vi "Ramp to Zero.vi"(8 "error in (no error)":errorcluster, 11 "Instrument.1820 in":refnum<class "Instrument.Oxford1820.lvclass">) -> (0 "error out":errorcluster, 2 "Response":string, 3 "Instrument.1820 in":refnum<class "Instrument.Oxford1820.lvclass">)   [LabVIEW 2016, in "Instrument.Oxford1820.lvclass"]
uses:
  Instrument.Oxford1820.lvclass
  <instrlib>/Mercury iXX/Public/Libraries/Magnet/Controls/PSU Actions.ctl
  Typedefs/Instrument.Oxford1820.Commands-enum.ctl
  <instrlib>/Mercury iXX/Public/Libraries/Magnet.lvlib
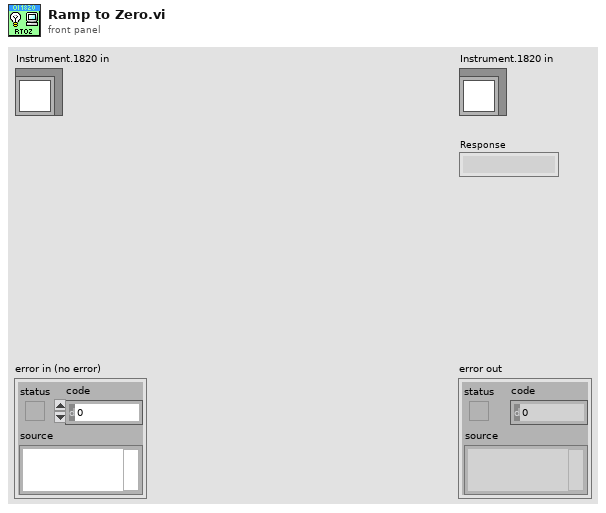
[diagram p1: front panel]
types:
  T1 = typedef "Instrument.Oxford1820.lvclass/Instrument.Oxford1820.Commands-enum.ctl" = enum16{"setAction", "setTarget", "setSwitchHeat", "setLambda", "setFillMode", "setNeedleValve", "setMagnetField", "getStatus", "getTarget", "getSwitchHeat", "getPSUField", "newcommand", "getMagnetField"}
  T2 = typedef "Mercury iXX.lvlib/Magnet.lvlib/PSU Actions.ctl" = string
  T3 = cluster{"Holding":bool, "Ramp to Setpoint":bool, "Ramp to Zero":bool, "Clamp":bool}
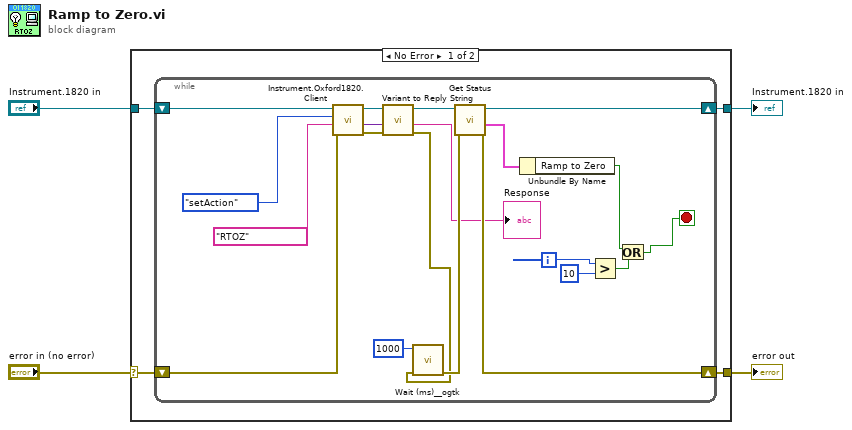
[diagram p0: block diagram]
diagram:
  n1 = case shown="No Error" "error in (no error)" {
    selector: "error in (no error)" -> [w7 w30]
    tunnel: [w5 w30] -> w3
    tunnel: [w6 w29] -> w1
    tunnel: "Instrument.1820 in" -> [w8 w29]
    frame No Error {
      n2 = while {
        shift-right: [w23] -> w6
        shift-left: w8 -> [w20]
        shift-right: [w21] -> w5
        shift-left: w7 -> [w26]
        i -> [w17]
        stop <- w15 stop-if-true
        n3 = call "Instrument.Oxford1820.Client.vi"("error in (no error)"=w26, "Data"=T2 "RTOZ" ("PSU Act Stat"), "Commands"=Instrument.Oxford1820.Commands-enum."setAction", "Instrument.1820 in"=w20) -> ("error out"=w9:errorcluster, "Data out"=w10:variant, "Instrument.1820 out"=w13:refnum<class "Instrument.Oxford1820.lvclass">)  [unwired: 5 in]
        n4 = call "Variant to Reply String.vi"("error in (no error)"=w9, "Data"=w10, "Instrument.1820 in"=w13) -> ("error out"=w12:errorcluster, "Reply"=→"Response":string, "Instrument.1820 out"=w11:refnum<class "Instrument.Oxford1820.lvclass">)  [unwired: 6 in]
        n5 = call <userlib>:"Wait (ms)__ogtk.vi"("error in (no error)"=w12, "milliseconds to wait"=u32 1000) -> ("error out"=w22:errorcluster)  [unwired: 8 in, 1 out]
        n6 = call "Get Status.vi"("error in (no error)"=w22, "Instrument.1820 in"=w11) -> ("error out"=w21:errorcluster, "Status"=w24:T3, "Instrument.1820 in"=w23:refnum<class "Instrument.Oxford1820.lvclass">)  [unwired: 6 in, 1 out]
        n7 = Unbundle By Name(w24) -> ("Ramp to Zero"=w16:bool)
        n8 = Greater?(x=w17, y=10) -> (0:w18:bool)
        n9 = Or(x=w16, y=w18) -> (x .or. y?=w15:bool)
      }
    }
    frame Error {
    }
  }
  "error out" <- w3
  "Instrument.1820 in" <- w1
